vi "GA Buf IO.vi"(4 "segNum":i32, 5 "FifoIndex":i16, 6 "doValue":u16, 7 "doMask":u16, 8 "error in (no error)":errorcluster caption="错误输入（无错误）", 9 "nCardIndex":u16, 10 "nDoType":u16, 11 "nCrdNum":i16) -> (0 "error out":errorcluster caption="错误输出", 3 "function return":i32)   [LabVIEW 2015, in "GAS.lvlib"]
doc: "extern \"C\" __declspec(dllimport) int GA_BufIO(short nCrdNum,unsigned short nDoType,unsigned short nCardIndex,unsigned short doMask,unsigned short doValue,short FifoIndex=0,long segNum = 0);"
uses:
  <userlib>/BP_GAS/GAS.lvlib
  <userlib>/BP_GAS/GAS.dll
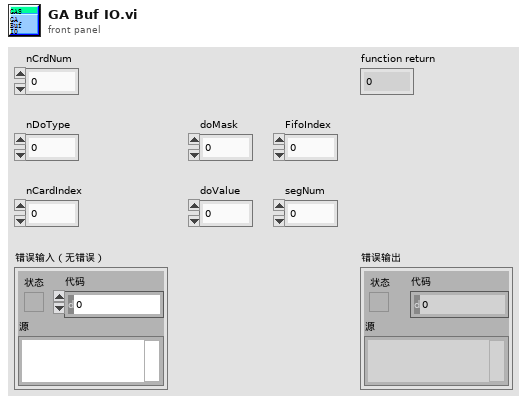
[diagram p1: front panel]
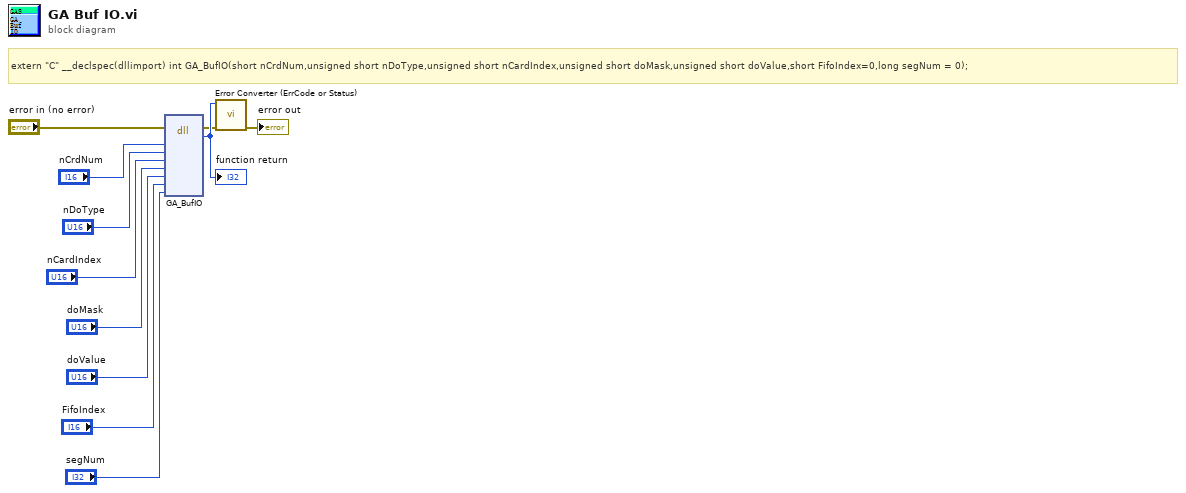
[diagram p0: block diagram]
diagram:
  # "extern \"C\" __declspec(dllimport) int GA_BufIO(short nCrdNum,unsigned short nDoType,unsigned short nCardIndex,unsigned short doMask,unsigned short doValue,short FifoIndex=0,long segNum = 0);"
  n1 = dll-call lib="E:/Program Files (x86)/National Instruments/LabVIEW 2015/user.lib/BP_GAS/GAS.*" fn="GA_BufIO"(error in="error in (no error)", "nCrdNum"="nCrdNum", "nDoType"="nDoType", "nCardIndex"="nCardIndex", "doMask"="doMask", "doValue"="doValue", "FifoIndex"="FifoIndex", "segNum"="segNum") -> (error out=w2:errorcluster, w11:i32)  [unwired: 9 in, 1 out]
  "function return" <- w11
  n2 = call "Error Converter (ErrCode or Status).vi"("error in (no error)"=w2, "error code"=w11) -> ("error out"=→"error out":errorcluster)  [unwired: 9 in]
